vi "serialcom.vi"() -> ()   [LabVIEW 2017]
uses:
  <vilib>/Instr/_visa.llb/VISA Configure Serial Port (Instr).vi
panel:
  in  "Play Music":bool
  out "Temperature Chart":dbl(graph)
  out "Thermometer":dbl(slide) scale=0.0..100.0
  out "Current temperature":dbl
  in  "Read":bool
  in  "Stop bits":u16(ring)=10 items=["1.0"=10, "1.5"=15, "2.0"=20]
  in  "Parity":enum16{"None", "Odd", "Even", "Mark", "Space"}(ring)
  in  "Data bits":u16=8 min=5 max=8 step=1
  in  "COM PORT":refnum<visa-resource-name>
  in  "Stop":bool
  in  "Baud rate":i32
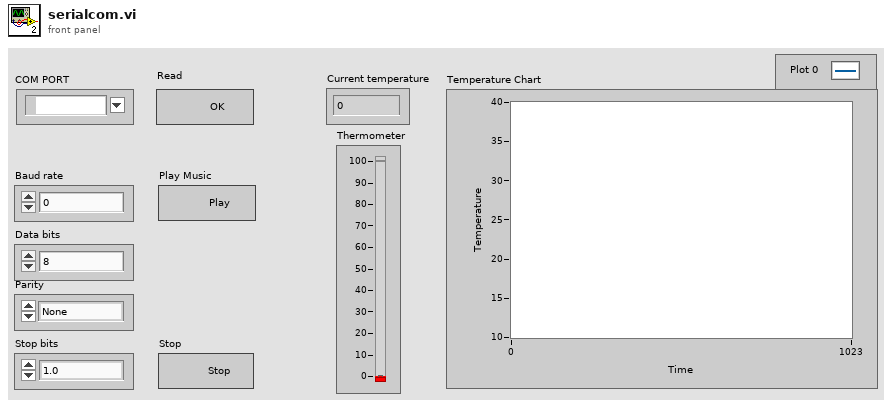
[diagram p1: front panel]
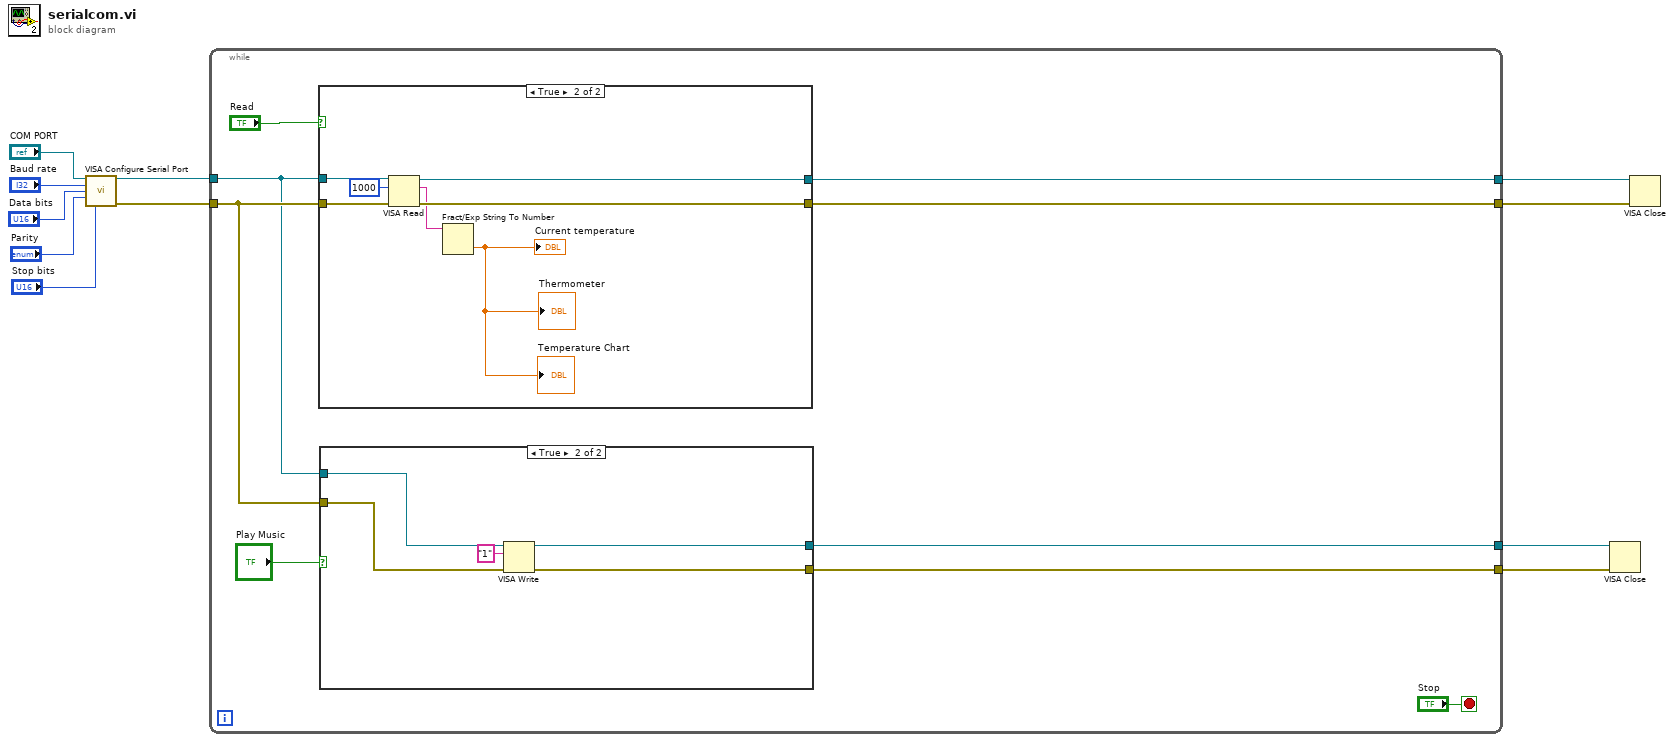
[diagram p0: block diagram]
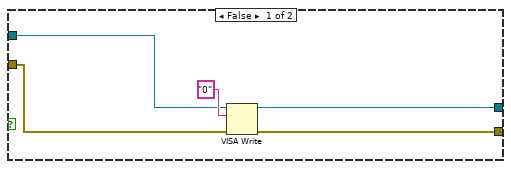
[diagram p2: hidden frame]
diagram:
  n1 = call-poly "VISA Configure Serial Port"("VISA resource name"="COM PORT", "baud rate (9600)"="Baud rate", "data bits (8)"="Data bits", "parity (0:none)"="Parity", "stop bits (10: 1 bit)"="Stop bits") -> ("VISA resource name out"=w11:refnum<visa-resource-name>, "error out"=w4:errorcluster)  [unwired: 9 in]
  n2 = while {
    tunnel: w4 -> [w16]
    tunnel: [w19] -> w5
    tunnel: [w18] -> w6
    tunnel: w11 -> [w15]
    tunnel: [w14] -> w2
    tunnel: [w13] -> w1
    stop <- "Stop" stop-if-true
    n3 = case shown="True" "Read" {
      tunnel: w16 -> [w31 w39]
      tunnel: [w31 w38] -> w19
      tunnel: [w32 w37] -> w18
      tunnel: w15 -> [w32 w36]
      frame False {
      }
      frame True {
        n4 = VISA Read(VISA resource name=w36, byte count=u32 1000, error in (no error)=w39) -> (VISA resource name out=w37:refnum<visa-resource-name>, read buffer=w34:string, error out=w38:errorcluster)  [unwired: 1 out]
        n5 = Fract/Exp String To Number(string=w34) -> (number=→"Current temperature" →"Thermometer" →"Temperature Chart":dbl)  [unwired: 3 in, 1 out]
      }
    }
    n6 = case shown="True" "Play Music" {
      tunnel: w16 -> [w21 w30]
      tunnel: w15 -> [w22 w29]
      tunnel: [w23 w27] -> w14
      tunnel: [w24 w26] -> w13
      frame False {
        n7 = VISA Write(VISA resource name=w22, write buffer="0", error in (no error)=w21) -> (VISA resource name out=w23:refnum<visa-resource-name>, error out=w24:errorcluster)  [unwired: 1 out]
      }
      frame True {
        n8 = VISA Write(VISA resource name=w29, write buffer="1", error in (no error)=w30) -> (VISA resource name out=w27:refnum<visa-resource-name>, error out=w26:errorcluster)  [unwired: 1 out]
      }
    }
  }
  n9 = VISA Close(VISA resource name=w2, error in (no error)=w1) -> ()  [unwired: 1 out]
  n10 = VISA Close(VISA resource name=w6, error in (no error)=w5) -> ()  [unwired: 1 out]
